vi "Read VISA Port.vi"(8 "error in (no error)":errorcluster, 11 "RS232_Device in":refnum<class "RS232_Device.lvclass">) -> (0 "error out":errorcluster, 2 "VISA Port":string, 3 "RS232_Device out":refnum<class "RS232_Device.lvclass">)   [LabVIEW 2023, in "RS232_Device.lvclass"]
uses:
  RS232_Device.lvclass
  RS232_Device.lvclass/RS232_Device.ctl
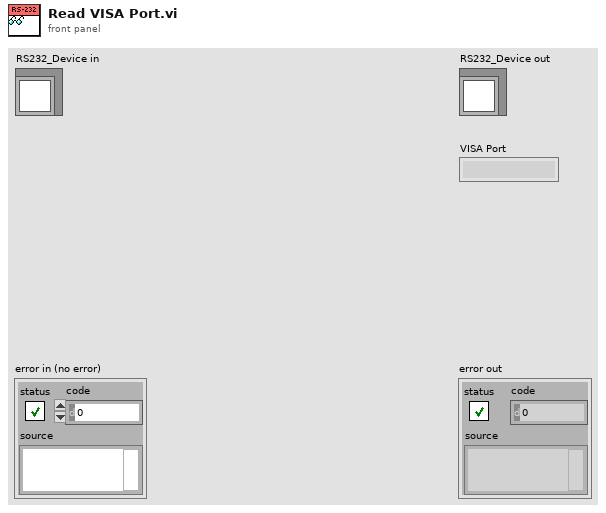
[diagram p1: front panel]
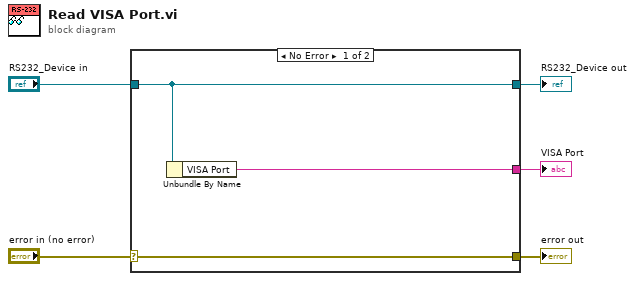
[diagram p0: block diagram]
diagram:
  n1 = case shown="No Error" "error in (no error)" {
    selector: "error in (no error)" -> [w8 w9]
    tunnel: [w8 w9] -> w4
    tunnel: [w7 w10] -> w2
    tunnel: "RS232_Device in" -> [w7 w10]
    tunnel: [w6 _] -> w1
    frame No Error {
      n2 = Unbundle By Name(w7) -> ("VISA Port"=w6:string)
    }
    frame Error {
    }
  }
  "error out" <- w4
  "RS232_Device out" <- w2
  "VISA Port" <- w1
